vi "RobotNTViewer.vi"() -> ()   [LabVIEW 2016]
panel:
  in  "NT Entries":string(tree)
  in  "Tab Control":enum32{"Drivetrain", "Shooter", "Power Data"}(tab)
  in  "driveGraphSeconds":dbl=60.0 caption="seconds to display"
  out "leftPosSet":dbl
  out "rightPosSet":dbl
  out "centerPosSet":dbl
  out "leftVelSet":dbl
  out "rightVelSet":dbl
  out "centerVelSet":dbl
  out "Drive Graph":waveform(dbl)[](graph)
  out "frontTraction":bool
  out "rearTraction":bool
  out "leftDriveVel":dbl
  out "leftDrivePos":dbl
  out "centerDriveVel":dbl
  out "centerDrivePos":dbl
  out "rightDriveVel":dbl
  out "rightDrivePos":dbl
  out "robotYaw":dbl
  in  "freezeDriveVel":bool
  out "leftOut":dbl
  out "rightOut":dbl
  out "centerOut":dbl
  in  "driveDisplay":T1(ring) caption="Display Mode"
  in  "FreezeShooter":bool caption="Freeze"
  out "Shooter graph":waveform(dbl)[](graph)
  out "shooterOutput":dbl
  out "shooterOn":bool
  out "shooterSetpoint":dbl
  out "shooterRPM":dbl
  out "augerCurrent":dbl
  out "intakeCurrent":dbl
  out "shooterCurrent":dbl
  out "hangarCurrent":dbl
  in  "Freeze Current":bool
  out "Amperage":waveform(dbl)[](graph)
  out "totalCurrent":dbl
  out "centerCurrent":dbl[](array[numeric])
  out "rightCurrent":dbl[](array[numeric])
  out "leftCurrent":dbl[](array[numeric])
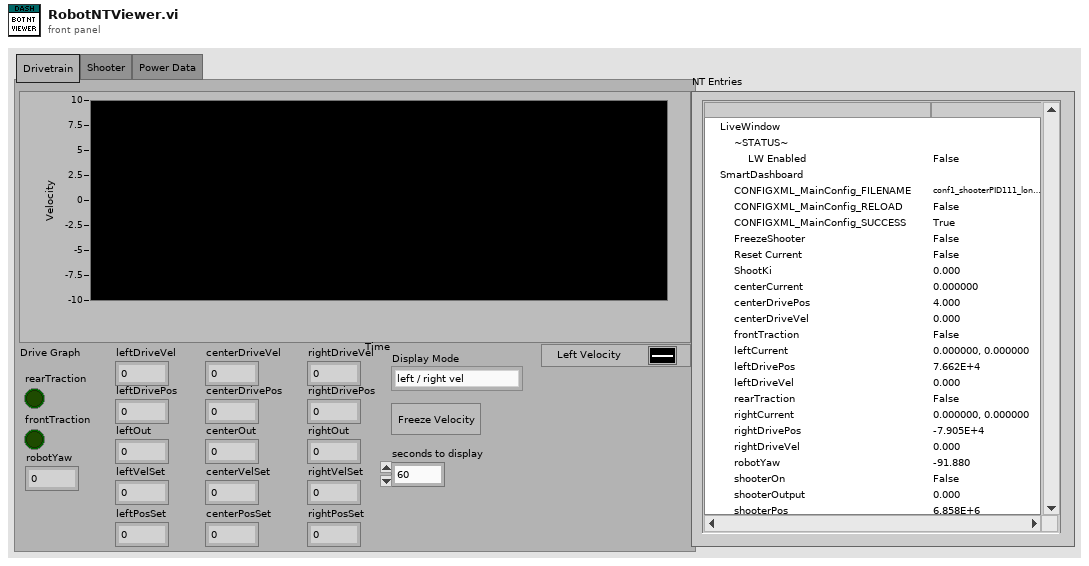
[diagram p1: front panel]
types:
  T1 = enum16{"left / right vel", "left / right pos", "center vel", "center pos"}
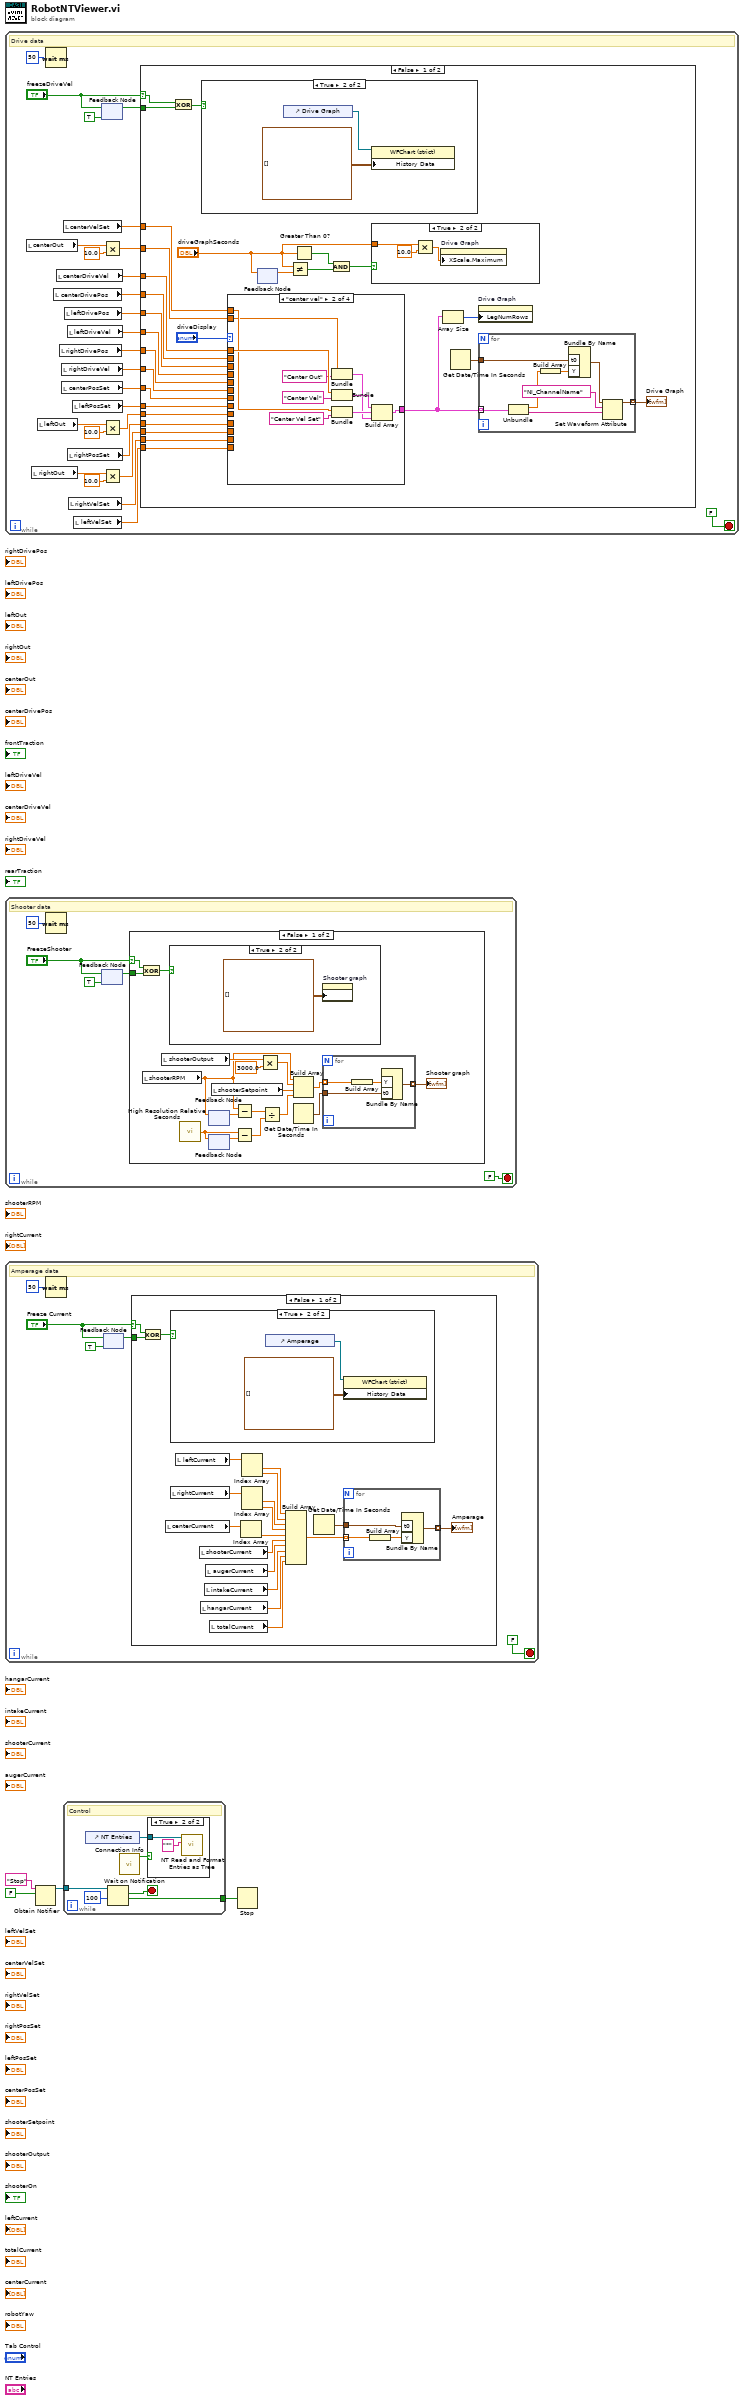
[diagram p0: block diagram]
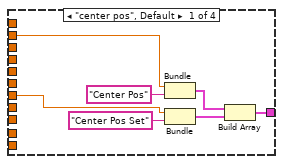
[diagram p3: hidden frame]
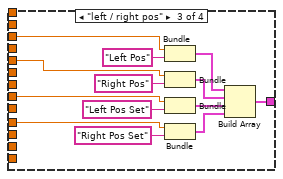
[diagram p4: hidden frame]
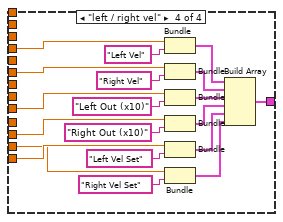
[diagram p5: hidden frame]
diagram:
  n1 = while {
    stop <- FALSE stop-if-true
    # "Drive data"
    n2 = local read "centerOut"() -> (w24:dbl)
    n3 = local read "rightOut"() -> (w23:dbl)
    n4 = local read "leftOut"() -> (w20:dbl)
    n5 = Wait (ms)(milliseconds to wait=u32 50) -> ()  [unwired: 1 out]
    n6 = local read "centerDrivePos"() -> (w11:dbl)
    n7 = local read "centerDriveVel"() -> (w14:dbl)
    n8 = local read "rightDrivePos"() -> (w12:dbl)
    n9 = local read "rightDriveVel"() -> (w18:dbl)
    n10 = local read "centerPosSet"() -> (w8:dbl)
    n11 = local read "centerVelSet"() -> (w6:dbl)
    n12 = local read "leftDrivePos"() -> (w13:dbl)
    n13 = local read "leftDriveVel"() -> (w19:dbl)
    n14 = local read "rightPosSet"() -> (w9:dbl)
    n15 = local read "rightVelSet"() -> (w5:dbl)
    n16 = local read "leftPosSet"() -> (w10:dbl)
    n17 = local read "leftVelSet"() -> (w7:dbl)
    n18 = feedback #1(TRUE ("Freeze Current")) -> (w27:bool)
    n19 = feedback-in #1("freezeDriveVel") -> ()
    n20 = Multiply(x=w24, y=10.0) -> (x*y=w15:dbl)
    n21 = Multiply(x=w20, y=10.0) -> (x*y=w17:dbl)
    n22 = Multiply(x=w23, y=10.0) -> (x*y=w16:dbl)
    n23 = case shown="False" "freezeDriveVel" {
      selector: "freezeDriveVel" -> [w57 _]
      tunnel: w27 -> [w56 _]
      tunnel: w19 -> [w44 _]
      tunnel: w18 -> [w45 _]
      tunnel: w17 -> [w46 _]
      tunnel: w16 -> [w47 _]
      tunnel: w15 -> [w49 _]
      tunnel: w14 -> [w48 _]
      tunnel: w13 -> [w50 _]
      tunnel: w12 -> [w51 _]
      tunnel: w11 -> [w52 _]
      tunnel: w10 -> [w41 _]
      tunnel: w9 -> [w40 _]
      tunnel: w8 -> [w39 _]
      tunnel: w7 -> [w38 _]
      tunnel: w6 -> [w37 _]
      tunnel: w5 -> [w36 _]
      frame False {
        n24 = Exclusive Or(1:w56, 2:w57) -> (0:w55:bool)
        n25 = case shown="True" w55 {
          frame False {
          }
          frame True {
            n26 = control-ref of="Drive Graph"() -> (w111:refnum<vi>)
            n27 = property class="WFChart (strict)"(reference=w111, "History Data"=waveform(dbl)[][] []) -> ()  [unwired: 1 in, 2 out]
          }
        }
        n28 = case shown="\"center vel\"" "driveDisplay" {
          tunnel: w52 -> [w68 _ _ _]
          tunnel: w51 -> [_ _ w87 _]
          tunnel: w50 -> [_ _ w89 _]
          tunnel: w49 -> [_ w70 _ _]
          tunnel: w48 -> [_ w76 _ _]
          tunnel: w47 -> [_ _ _ w101]
          tunnel: w46 -> [_ _ _ w102]
          tunnel: w45 -> [_ _ _ w103]
          tunnel: w44 -> [_ _ _ w104]
          tunnel: [w65 w77 w85 w98] -> w43
          tunnel: w41 -> [_ _ w80 _]
          tunnel: w40 -> [_ _ w79 _]
          tunnel: w39 -> [w62 _ _ _]
          tunnel: w38 -> [_ _ _ w93]
          tunnel: w37 -> [_ w74 _ _]
          tunnel: w36 -> [_ _ _ w92]
          frame "center pos", Default {
            n29 = Bundle("centerDrivePos"=w68, "Center Pos") -> (w66:cluster{"centerDrivePos":dbl, string})  [unwired: 1 in]
            n30 = Bundle("centerPosSet"=w62, "Center Pos Set") -> (w63:cluster{"centerPosSet":dbl, string})  [unwired: 1 in]
            n31 = Build Array(w66, w63) -> (w65:cluster{"centerPosSet":dbl, string}[])
          }
          frame "center vel" {
            n32 = Bundle(w70, "Center Out") -> (w69:cluster{dbl, string})  [unwired: 1 in]
            n33 = Bundle("centerDriveVel"=w76, "Center Vel") -> (w71:cluster{"centerDriveVel":dbl, string})  [unwired: 1 in]
            n34 = Bundle("centerVelSet"=w74, "Center Vel Set") -> (w73:cluster{"centerVelSet":dbl, string})  [unwired: 1 in]
            n35 = Build Array(w71, w73, w69) -> (w77:cluster{"centerVelSet":dbl, string}[])
          }
          frame "left / right pos" {
            n36 = Bundle("leftDrivePos"=w89, "Left Pos") -> (w90:cluster{"leftDrivePos":dbl, string})  [unwired: 1 in]
            n37 = Bundle("rightDrivePos"=w87, "Right Pos") -> (w86:cluster{"rightDrivePos":dbl, string})  [unwired: 1 in]
            n38 = Bundle("leftPosSet"=w80, "Left Pos Set") -> (w81:cluster{"leftPosSet":dbl, string})  [unwired: 1 in]
            n39 = Bundle("rightPosSet"=w79, "Right Pos Set") -> (w82:cluster{"rightPosSet":dbl, string})  [unwired: 1 in]
            n40 = Build Array(w90, w86, w81, w82) -> (w85:cluster{"rightPosSet":dbl, string}[])
          }
          frame "left / right vel" {
            n41 = Bundle("leftDriveVel"=w104, "Left Vel") -> (w109:cluster{"leftDriveVel":dbl, string})  [unwired: 1 in]
            n42 = Bundle("rightDriveVel"=w103, "Right Vel") -> (w107:cluster{"rightDriveVel":dbl, string})  [unwired: 1 in]
            n43 = Bundle(w102, "Left Out (x10)") -> (w99:cluster{dbl, string})  [unwired: 1 in]
            n44 = Bundle(w101, "Right Out (x10)") -> (w100:cluster{dbl, string})  [unwired: 1 in]
            n45 = Bundle("leftVelSet"=w93, "Left Vel Set") -> (w94:cluster{"leftVelSet":dbl, string})  [unwired: 1 in]
            n46 = Bundle("rightVelSet"=w92, "Right Vel Set") -> (w95:cluster{"rightVelSet":dbl, string})  [unwired: 1 in]
            n47 = Build Array(w109, w107, w99, w100, w94, w95) -> (w98:cluster{"rightVelSet":dbl, string}[])
          }
        }
        n48 = feedback-in #2("driveGraphSeconds") -> ()
        n49 = feedback #2() -> (w32:dbl)  [unwired: 1 in]
        n50 = Not Equal?(x="driveGraphSeconds", y=w32) -> (x != y?=w35:bool)
        n51 = Greater Than 0?(x="driveGraphSeconds") -> (x > 0?=w34:bool)
        n52 = And(x=w34, y=w35) -> (x .and. y?=w33:bool)
        n53 = case shown="True" w33 {
          tunnel: "driveGraphSeconds" -> [_ w61]
          frame False {
          }
          frame True {
            n54 = Multiply(x=w61, y=10.0) -> (x*y=w59:dbl)
            n55 = property on="Drive Graph" class="WFChart (strict)"("XScale.Maximum"=w59) -> ()  [unwired: 2 in, 2 out]
          }
        }
        n56 = Array Size(array=w43) -> (size(s)=w42:i32)
        n57 = Get Date/Time In Seconds() -> (seconds since 1Jan1904=w58:timestamp)
        n58 = property on="Drive Graph" class="WFChart (strict)"("LegNumRows"=w42) -> ()  [unwired: 2 in, 2 out]
        n59 = for {
          tunnel: w58 -> [w120]
          tunnel: [w118] -> w54 mode=indexing
          tunnel: w43 -> [w116] mode=indexing
          n60 = Unbundle(w116) -> ("rightVelSet"=w115:dbl, w113:string)
          n61 = Build Array(w115) -> (w114:dbl[])
          n62 = Bundle By Name("t0"=w120, "Y"=w114) -> (w119:waveform(dbl))  [unwired: 1 in]
          n63 = Set Waveform Attribute(5:w113, 6:"NI_ChannelName" ("name"), 7:w119) -> (3:w118:waveform(dbl))  [unwired: 1 in, 2 out]
        }
        "Drive Graph" <- w54
      }
      frame True {
      }
    }
  }
  n64 = while {
    stop <- FALSE stop-if-true
    # "Shooter data"
    n65 = Wait (ms)(milliseconds to wait=u32 50) -> ()  [unwired: 1 out]
    n66 = feedback-in #3("FreezeShooter") -> ()
    n67 = feedback #3(TRUE ("FreezeShooter")) -> (w121:bool)
    n68 = case shown="False" "FreezeShooter" {
      selector: "FreezeShooter" -> [w128 _]
      tunnel: w121 -> [w127 _]
      frame False {
        n69 = Exclusive Or(1:w127, 2:w128) -> (0:w126:bool)
        n70 = local read "shooterRPM"() -> (w135:dbl)
        n71 = local read "shooterOutput"() -> (w140:dbl)
        n72 = case shown="True" w126 {
          frame False {
          }
          frame True {
            n73 = property on="Shooter graph" class="WFChart (strict)"("History Data"=waveform(dbl)[][] []) -> ()  [unwired: 2 in, 2 out]
          }
        }
        n74 = call <vilib>:"High Resolution Relative Seconds.vi"() -> ("relative seconds"=w132:dbl)
        n75 = feedback-in #4(w135) -> ()
        n76 = feedback #4() -> (w134:dbl)  [unwired: 1 in]
        n77 = feedback-in #5(w132) -> ()
        n78 = feedback #5() -> (w131:dbl)  [unwired: 1 in]
        n79 = local read "shooterSetpoint"() -> (w142:dbl)
        n80 = Subtract(x=w135, y=w134) -> (x-y=w133:dbl)
        n81 = Subtract(x=w132, y=w131) -> (x-y=w130:dbl)
        n82 = Multiply(x=w140, y=3000.0) -> (x*y=w141:dbl)
        n83 = Divide(x=w133, y=w130) -> (x/y=w129:dbl)
        n84 = Build Array(w135, w141, w142, w129) -> (w138:dbl[])
        n85 = Get Date/Time In Seconds() -> (seconds since 1Jan1904=w137:timestamp)
        n86 = for {
          tunnel: w138 -> [w147] mode=indexing
          tunnel: w137 -> [w145]
          tunnel: [w144] -> w136 mode=indexing
          n87 = Build Array(w147) -> (w146:dbl[])
          n88 = Bundle By Name("Y"=w146, "t0"=w145) -> (w144:waveform(dbl))  [unwired: 1 in]
        }
        "Shooter graph" <- w136
      }
      frame True {
      }
    }
  }
  n89 = while {
    stop <- FALSE stop-if-true
    # "Amperage data"
    n90 = Wait (ms)(milliseconds to wait=u32 50) -> ()  [unwired: 1 out]
    n91 = feedback-in #6("Freeze Current") -> ()
    n92 = feedback #6(TRUE ("Freeze Current")) -> (w149:bool)
    n93 = case shown="False" "Freeze Current" {
      selector: "Freeze Current" -> [w159 _]
      tunnel: w149 -> [w158 _]
      frame False {
        n94 = Exclusive Or(1:w158, 2:w159) -> (0:w157:bool)
        n95 = local read "centerCurrent"() -> (w165:dbl[])
        n96 = case shown="True" w157 {
          frame False {
          }
          frame True {
            n97 = control-ref of="Amperage"() -> (w173:refnum<vi>)
            n98 = property class="WFChart (strict)"(reference=w173, "History Data"=waveform(dbl)[][] []) -> ()  [unwired: 1 in, 2 out]
          }
        }
        n99 = local read "rightCurrent"() -> (w164:dbl[])
        n100 = local read "leftCurrent"() -> (w163:dbl[])
        n101 = local read "shooterCurrent"() -> (w154:dbl)
        n102 = local read "hangarCurrent"() -> (w153:dbl)
        n103 = local read "intakeCurrent"() -> (w155:dbl)
        n104 = local read "augerCurrent"() -> (w156:dbl)
        n105 = local read "totalCurrent"() -> (w171:dbl)
        n106 = Index Array(array=w165) -> (element=w170:dbl)  [unwired: 1 in]
        n107 = Index Array(array=w163) -> (element #1=w166:dbl, element #2=w167:dbl)  [unwired: 2 in]
        n108 = Index Array(array=w164) -> (element #1=w168:dbl, element #2=w169:dbl)  [unwired: 2 in]
        n109 = Build Array(w166, w167, w168, w169, w170, w154, w156, w155, w153, w171) -> (w162:dbl[])
        n110 = Get Date/Time In Seconds() -> (seconds since 1Jan1904=w161:timestamp)
        n111 = for {
          tunnel: w162 -> [w176] mode=indexing
          tunnel: w161 -> [w177]
          tunnel: [w174] -> w160 mode=indexing
          n112 = Build Array(w176) -> (w175:dbl[])
          n113 = Bundle By Name("t0"=w177, "Y"=w175) -> (w174:waveform(dbl))  [unwired: 1 in]
        }
        "Amperage" <- w160
      }
      frame True {
      }
    }
  }
  n114 = Obtain Notifier(name (unnamed)="Stop", notification data type=FALSE ("notification")) -> (notifier out=w2:refnum<notifier>)  [unwired: 2 in, 2 out]
  n115 = while {
    tunnel: w2 -> [w179]
    tunnel: [w178] -> w1
    stop <- w183 stop-if-true
    # "Control"
    n116 = control-ref of="NT Entries"() -> (w180:refnum<vi>)
    n117 = Wait on Notification(notifier=w179, timeout in ms (-1)=100) -> (notification=w183:bool, timed out?=w178:bool)  [unwired: 2 in, 2 out]
    n118 = call <vilib>:"Connection Info.vi"() -> ("Connected"=w181:bool)  [unwired: 10 in, 1 out]
    n119 = case shown="True" w181 {
      tunnel: w180 -> [_ w185]
      frame False {
      }
      frame True {
        n120 = call <vilib>:"NT Read and Format Entries as Tree.vi"("Name Pattern"="*", "Tree Refnum"=w185) -> ()  [unwired: 8 in, 2 out]
      }
    }
  }
  n121 = Stop(stop? (T)=w1) -> ()
